vi "Transfer Teleop.vi"(11 "Buttons":bool[](array[boolean])) -> ()   [LabVIEW 2019]
panel:
  in  "Setpoint":dbl=0.2
  in  "Button Index":i32=4
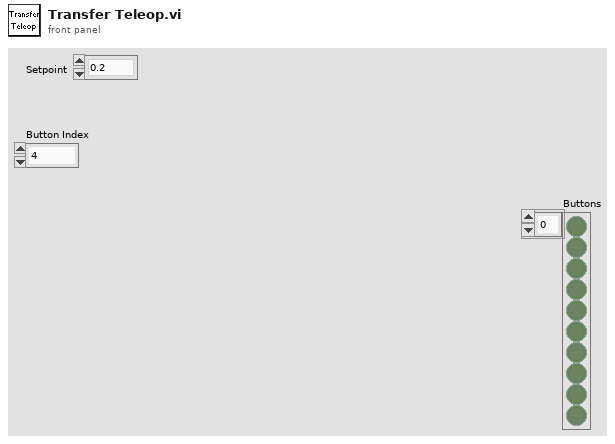
[diagram p1: front panel]
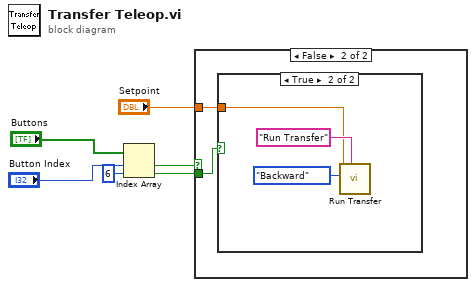
[diagram p0: block diagram]
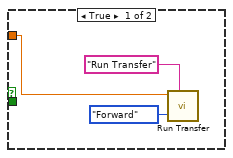
[diagram p2: hidden frame]
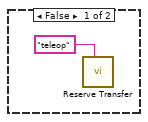
[diagram p3: hidden frame]
diagram:
  n1 = Index Array(array="Buttons", index #1="Button Index", index #2=6 ("index")) -> (element #1=w4:bool, element #2=w2:bool)
  n2 = case shown="False" w4 {
    tunnel: w2 -> [_ w11]
    tunnel: "Setpoint" -> [w7 w10]
    frame True {
      n3 = call "Run Transfer.vi"("Description"="Run Transfer", "Direction"=enum16{"Forward", "Backward"}."Forward", "Setpoint"=w7) -> ()  [unwired: 8 in, 1 out]
    }
    frame False {
      n4 = case shown="True" w11 {
        tunnel: w10 -> [_ w14]
        frame False {
          n5 = call "Reserve Transfer.vi"("Description"="teleop") -> ()  [unwired: 10 in, 1 out]
        }
        frame True {
          n6 = call "Run Transfer.vi"("Description"="Run Transfer", "Direction"=enum16{"Forward", "Backward"}."Backward", "Setpoint"=w14) -> ()  [unwired: 8 in, 1 out]
        }
      }
    }
  }
